vi "RSZVB Delete Balanced Port.vi"(8 "error in (no error)":errorcluster {"code" format="%.0x"}, 9 "Logical Port (1)":i32=1, 10 "Channel (1)":i32=1, 11 "VISA session":refnum<visa-resource-name>) -> (0 "error out":errorcluster {"code" format="%.0x"}, 3 "dup VISA session":refnum<visa-resource-name>)   [LabVIEW 2011]
doc: "This VI dissolves selected balanced port.\n\nRemote-control command(s):\nSOURce<Ch>:LPORt<log_port>:CLEar"
uses:
  _utility/RSZVB Global Data.vi
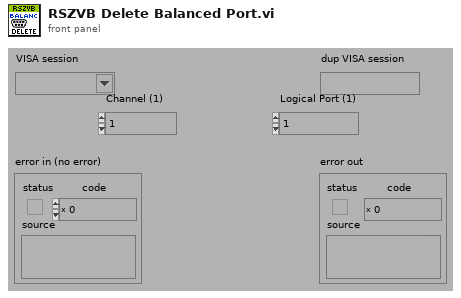
[diagram p1: front panel]
types:
  T1 = cluster{"Error Checking (T: On)":bool, "Installed Options":string[], "Data Valid?":bool, "Ports":i32, "Model":string[], "Option Checking (T: On)":bool}[]
  T2 = cluster{"Error Checking (T: On)":bool, "Installed Options":string[], "Data Valid?":bool, "Ports":i32, "Model":string[], "Option Checking (T: On)":bool}
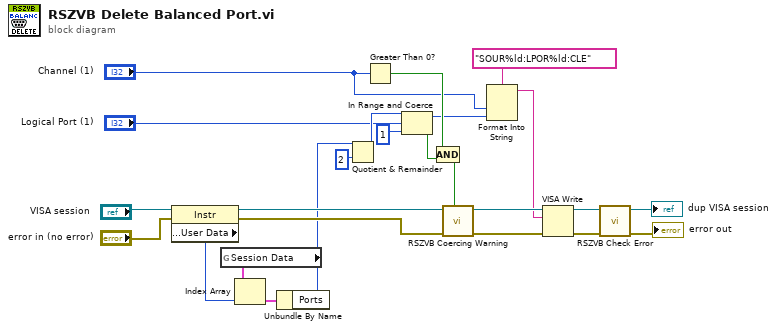
[diagram p0: block diagram]
diagram:
  n1 = property class="Instr"(reference="VISA session", error in="error in (no error)") -> (reference out=w13:refnum<visa-resource-name>, error out=w14:errorcluster, "General Settings:User Data"=w15:u32)
  n2 = global read "RSZVB Global Data.vi" "Session Data"() -> (w16:T1)
  n3 = Index Array(array=w16, index=w15) -> (element=w17:T2)
  n4 = Unbundle By Name(w17) -> ("Ports"=w2:i32)
  n5 = Quotient & Remainder(x=w2, y=2) -> (floor(x/y)=w9:i32)  [unwired: 1 out]
  n6 = Greater Than 0?(x="Channel (1)") -> (x > 0?=w18:bool)
  n7 = In Range and Coerce(upper limit=w9, x="Logical Port (1)", lower limit=1) -> (coerced(x)=w8:i32, In Range?=w11:bool)
  n8 = Compound Arithmetic op=AND(w18, w11) -> (w20:bool)
  n9 = call "RSZVB Coercing Warning.vi"("In Range?"=w20, "error in (no error)"=w14, "VISA session"=w13) -> ("error out"=w23:errorcluster, "dup VISA session"=w24:refnum<visa-resource-name>)  [unwired: 7 in]
  n10 = Format Into String(format string="SOUR%ld:LPOR%ld:CLE", "Channel (1)", w8) -> (resulting string=w19:string)  [unwired: 2 in, 1 out]
  n11 = VISA Write(VISA resource name=w24, write buffer=w19, error in (no error)=w23) -> (VISA resource name out=w21:refnum<visa-resource-name>, error out=w22:errorcluster)  [unwired: 1 out]
  n12 = call "RSZVB Check Error.vi"("error in (no error)"=w22, "VISA session"=w21) -> ("error out"=→"error out":errorcluster, "dup VISA session"=→"dup VISA session":refnum<visa-resource-name>)  [unwired: 8 in]
